vi "INST_PS_GET_VOLT-CURR-SET_LEVEL.vi"(0 "VISA session":refnum<visa-resource-name>, 11 "error in (no error)":errorcluster, 12 "line index":i32(ring) items=["1", "2", "3", "4", "ALL"], 13 "V/I":i32(ring) items=["VOLT", "CURR"], 14 "Use OPC(T)":bool) -> (3 "Voltage (0.0)":dbl[](array[numeric]) format="%.2p", 4 "dup VISA session":refnum<visa-resource-name>, 15 "error out":errorcluster)   [LabVIEW 2018]
doc: "This VI configures the DC voltage level the power supply attempts to generate.\n\nVer 3.0.0 supports the E36xx Model and The 6634B based on the GPIB address of idtATE [10-12]"
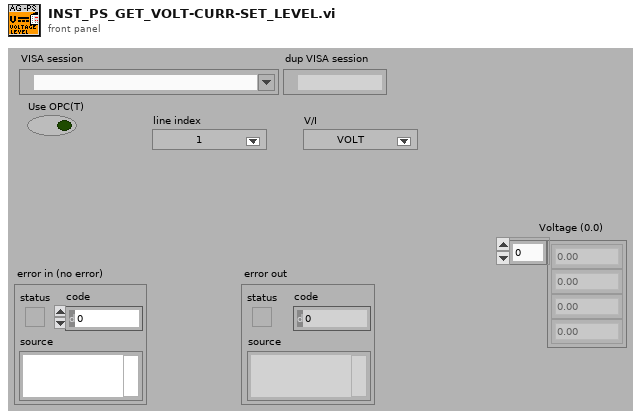
[diagram p1: front panel]
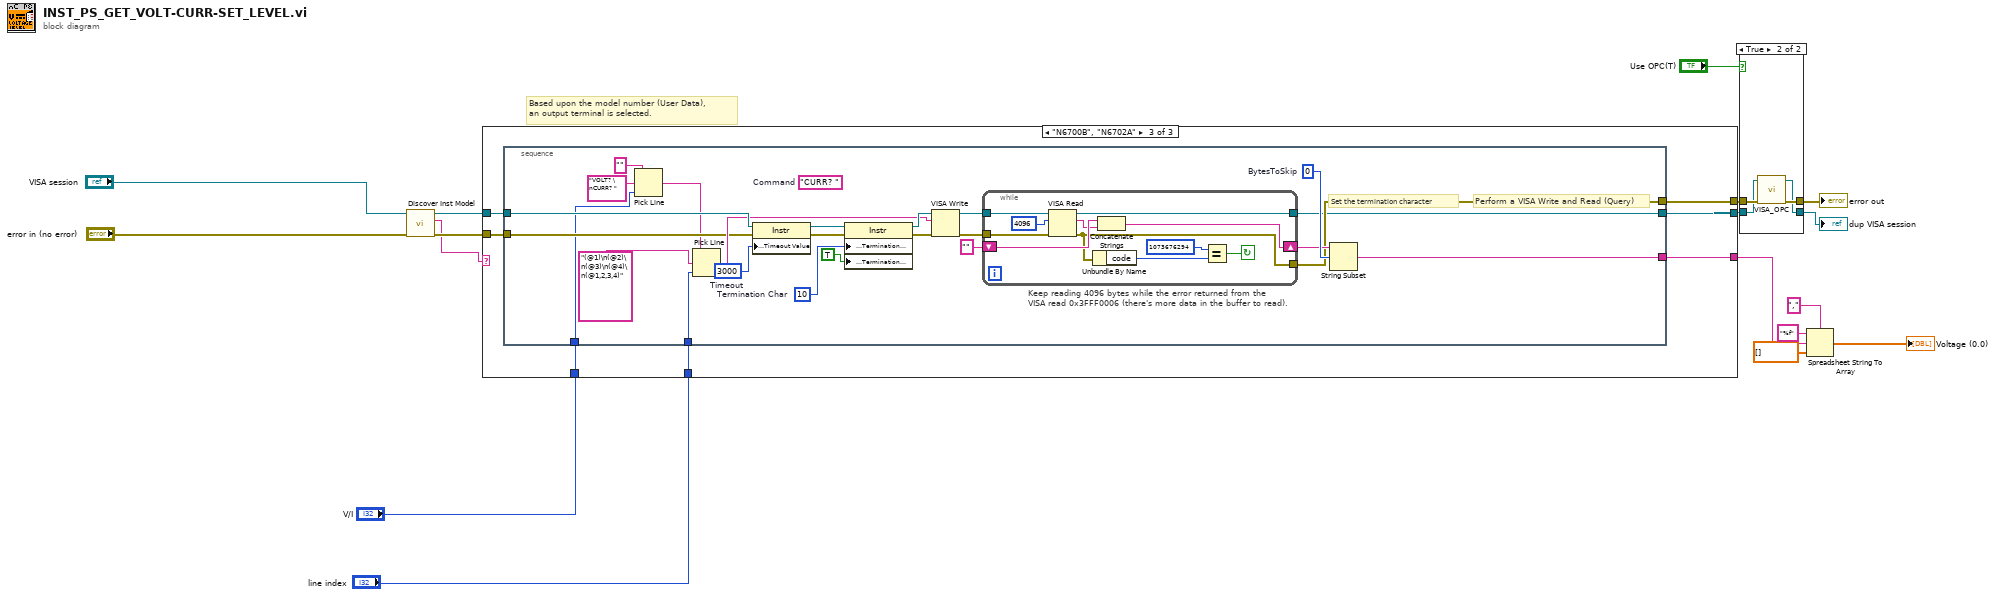
[diagram p0: block diagram]
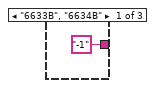
[diagram p2: hidden frame]
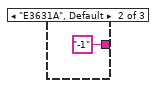
[diagram p3: hidden frame]
diagram:
  # "Based upon the model number (User Data), \nan output terminal is selected."
  n1 = call "Discover Inst Model.vi"("error in"="error in (no error)", "Session In"="VISA session") -> ("error out"=w13:errorcluster, "Model #"=w12:string, "Session Out"=w11:refnum<visa-resource-name>)  [unwired: 7 in]
  n2 = case shown="\"N6700B\", \"N6702A\"" w12 {
    tunnel: w13 -> [_ _ w23]
    tunnel: w11 -> [_ _ w26]
    tunnel: [_ _ w25] -> w10
    tunnel: [_ _ w24] -> w9
    tunnel: "line index" -> [_ _ w22]
    tunnel: ["-1" "-1" w21] -> w7
    tunnel: "V/I" -> [_ _ w20]
    frame "6633B", "6634B" {
    }
    frame "E3631A", Default {
    }
    frame "N6700B", "N6702A" {
      n3 = stacked-sequence {
        tunnel: w26 -> [w37]
        tunnel: [w47] -> w21
        tunnel: [w45] -> w25
        tunnel: [w35] -> w24
        tunnel: w23 -> [w31]
        tunnel: w22 -> [w34]
        tunnel: w20 -> [w27]
        frame #0 {
          (unwired) "CURR? "  # Command
          w49 = 0  # BytesToSkip
          w40 = u8 10  # Termination Char
          w36 = u32 3000  # Timeout
          # "Perform a VISA Write and Read (Query)"
          # "Keep reading 4096 bytes while the error returned from the\nVISA read 0x3FFF0006 (there's more data in the buffer to read)."
          # "Set the termination character"
          n4 = Pick Line(string ("")="", multi-line string="VOLT? \nCURR? ", line index=w27) -> (output string=w29:string)
          n5 = Pick Line(string ("")=w29, multi-line string="(@1)\n(@2)\n(@3)\n(@4)\n(@1,2,3,4)", line index=w34) -> (output string=w32:string)
          n6 = property class="Instr"(reference=w37, error in=w31, "General Settings:Timeout Value"=w36) -> (reference out=w41:refnum<visa-resource-name>, error out=w38:errorcluster)
          n7 = property class="Instr"(reference=w41, error in=w38, "Message Based Settings:Termination Character"=w40, "Message Based Settings:Termination Character Enable"=TRUE ("enable")) -> (reference out=w50:refnum<visa-resource-name>, error out=w39:errorcluster)
          n8 = VISA Write(VISA resource name=w50, write buffer=w32, error in (no error)=w39) -> (VISA resource name out=w43:refnum<visa-resource-name>, error out=w44:errorcluster)  [unwired: 1 out]
          n9 = while {
            tunnel: w43 -> [w58]
            shift-right: [w52] -> w48
            shift-left: "" -> [w57]
            tunnel: w44 -> [w55]
            tunnel: [w54] -> w45
            tunnel: [w51] -> w35
            stop <- w53 continue-if-true
            n10 = VISA Read(VISA resource name=w58, byte count=u32 4096 ("byte count (0)"), error in (no error)=w55) -> (VISA resource name out=w51:refnum<visa-resource-name>, read buffer=w56:string, error out=w54:errorcluster)  [unwired: 1 out]
            n11 = Unbundle By Name(w54) -> ("code"=w60:i32)
            n12 = Concatenate Strings(w57, w56) -> (w52:string)
            n13 = Equal?(x=1073676294, y=w60) -> (x = y?=w53:bool)
          }
          n14 = String Subset(string=w48, offset (0)=w49) -> (substring=w47:string)  [unwired: 1 out]
        }
      }
    }
  }
  n15 = case shown="True" "Use OPC(T)" {
    tunnel: w10 -> [w63 w66]
    tunnel: [w63 w67] -> w15
    tunnel: w9 -> [w62 w65]
    tunnel: [w62 w64] -> w16
    frame False {
    }
    frame True {
      n16 = call "VISA_OPC.vi"("error in"=w66, "Session In"=w65) -> ("error out"=w67:errorcluster, "Session Out"=w64:refnum<visa-resource-name>)  [unwired: 7 in, 1 out]
    }
  }
  "error out" <- w15
  "dup VISA session" <- w16
  n17 = Spreadsheet String To Array(delimiter (Tab)=",", format string="%f", spreadsheet string=w7, array type (2D Dbl)=dbl[] []) -> (array=→"Voltage (0.0)":dbl[])
